vi "subSave_AcquireFilterWheelInformation.vi"(3 "FWPosition":i32) -> (1 "FW text":string)   [LabVIEW 2015]
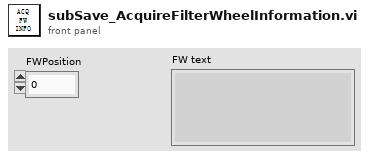
[diagram p1: front panel]
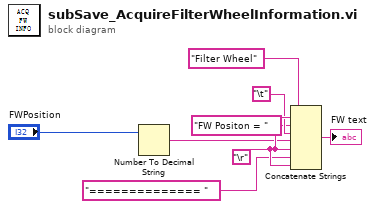
[diagram p0: block diagram]
diagram:
  w8 = "\r"
  n1 = Number To Decimal String(number="FWPosition") -> (decimal integer string=w3:string)  [unwired: 1 in]
  n2 = Concatenate Strings("Filter Wheel" ("string"), w8, "FW Positon = " ("string"), "\t", w3, w8, "============== " ("string"), w8) -> (→"FW text":string)
